vi "Definition.vi"(11 "NewEntityTemplate":refnum<class "MoarDemo.lvclass">) -> (2 "Entity Definition":refnum<class "Type.lvclass">[](array[class]))   [LabVIEW 2020, in "tests.lvlib" / "MoarDemo.lvclass"]
uses:
  MoarDemo.lvclass
  <vilib>/IlluminatedG/IG Conditum Base/Conditum/Columns/Type/Type.lvclass
  <vilib>/IlluminatedG/IG Conditum Base/Conditum/Columns/Integer/Integer.lvclass
  C:/Program Files (x86)/National Instruments/LabVIEW 2020/vi.lib/IlluminatedG/IG Conditum Base/Conditum/Columns/Type/Type.lvclass
  MoarDemo.lvclass/MoarDemo.ctl
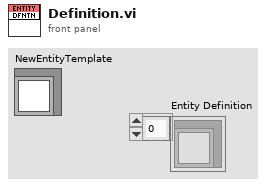
[diagram p1: front panel]
types:
  T1 = typedef "tests.lvlib/MoarDemo.lvclass/Columns.ctl" = cluster{"<Placeholder>":refnum<class "Integer.lvclass">}
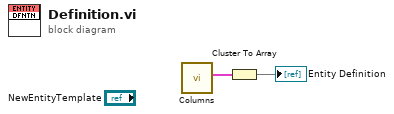
[diagram p0: block diagram]
diagram:
  n1 = call "Columns.vi"() -> ("Columns"=w2:T1)  [unwired: 11 in]
  n2 = Cluster To Array(cluster=w2) -> (array=→"Entity Definition":refnum<class "Integer.lvclass">[])
